vi "Polling.vi"() -> ()   [LabVIEW 2012]
panel:
  out "Current Time":timestamp
  in  "Time Check":bool
  out "Iteration":i32
  in  "Stop":bool
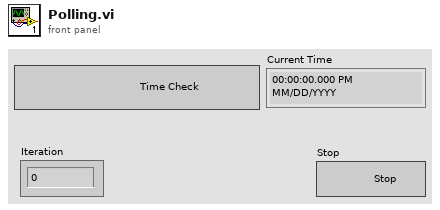
[diagram p1: front panel]
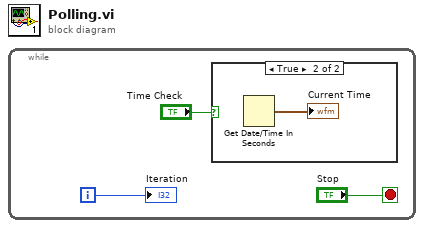
[diagram p0: block diagram]
diagram:
  n1 = while {
    i -> [w2]
    stop <- "Stop" stop-if-true
    n2 = case shown="True" "Time Check" {
      frame False {
      }
      frame True {
        n3 = Get Date/Time In Seconds() -> (seconds since 1Jan1904=→"Current Time":timestamp)
      }
    }
    "Iteration" <- w2
  }
